vi "get-childs-tags-by-tag.vi"(8 "error in (no error)":errorcluster, 9 "tag":string, 11 "CANtable in":refnum<class "bAPPdata.lvclass">) -> (0 "error out":errorcluster, 1 "child.tags":string[](array[string]), 3 "CANtable out":refnum<class "bAPPdata.lvclass">)   [LabVIEW 2015, in "bAPPdata.lvclass"]
uses:
  bAPPdata.lvclass
  bAPPdata.lvclass/bAPPdata.ctl
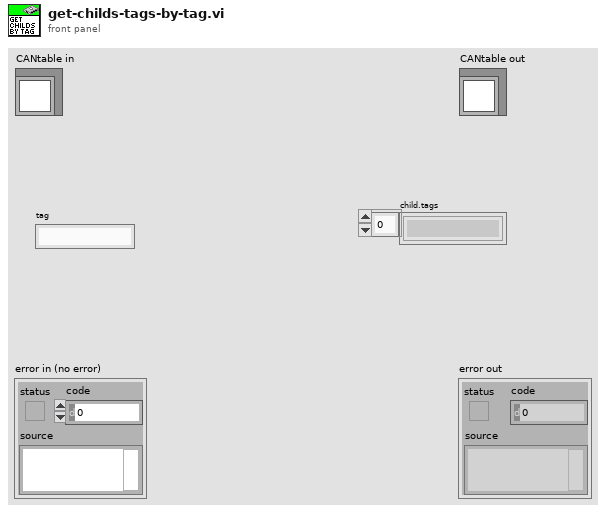
[diagram p1: front panel]
types:
  T1 = typedef "bAPPdata.lvclass/table-data.ctl" = T2[]
  T2 = typedef "bAPPdata.lvclass/table-contents.ctl" = cluster{"id":u32, "tag":string, "frame.type":T3, "last.frame":T4, "tMsgData":T6, "child.tags":string[], "bit-payload":bool[]}
  T3 = typedef "frame.type.ctl" = enum16{"FRAME NOT DEFINED", "DUT OUTPUT FRAME", "DUT INPUT FRAME"}
  T4 = typedef "XNET Frame CAN.ctl" = cluster{"timestamp":timestamp, "payload":u8[], "identifier":u32, "type":T5, "extended?":bool, "echo?":bool}
  T5 = typedef "XNET Frame Type CAN.ctl" = u8
  T6 = typedef "nMsgData.ctl" = cluster{"dwID":u32, "count":u32, "dwCycleTime":dbl, "dwTime":dbl, "new msg":bool}
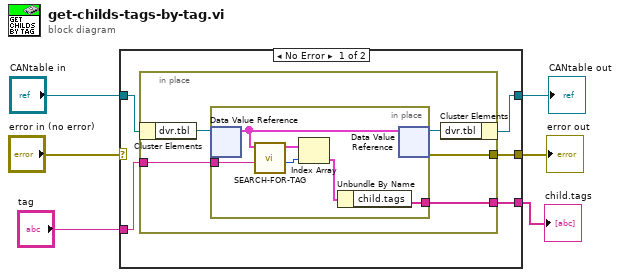
[diagram p0: block diagram]
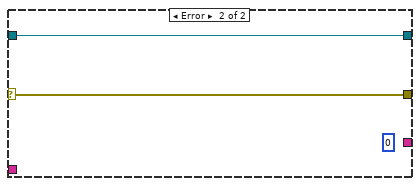
[diagram p2: hidden frame]
diagram:
  n1 = case shown="No Error" "error in (no error)" {
    selector: "error in (no error)" -> [_ w24]
    tunnel: [w9 w24] -> w5
    tunnel: [w10 w23] -> w3
    tunnel: "CANtable in" -> [w11 w23]
    tunnel: "tag" -> [w8 _]
    tunnel: [w7 _] -> w1
    frame No Error {
      n2 = in-place {
        in-place-border: [w14] -> w9
        in-place-border: w8 -> [w13]
        in-place-border: [w12] -> w7
        n3 = in-place-cluster #1(w11) -> ("dvr.tbl"=w16:refnum<data-value>)
        n4 = in-place {
          in-place-border: w13 -> [w18]
          in-place-border: [w17] -> w12
          n5 = in-place-dvr #2(w16) -> (w22:T1)  [unwired: 1 out]
          n6 = call "SEARCH-FOR-TAG.vi"("tag"=w18, "tbl.list"=w22) -> ("idx"=w21:i32, "tbl.list out"=w19:T2[])  [unwired: 8 in]
          n7 = Index Array(array=w19, index=w21) -> (element=w20:T2)
          n8 = Unbundle By Name(w20) -> ("child.tags"=w17:string[])
          n9 = in-place-dvr #2(w22) -> (w15:refnum<data-value>, w14:errorcluster)
        }
        n10 = in-place-cluster #1("dvr.tbl"=w15) -> (w10:refnum<class "bAPPdata.lvclass">)
      }
    }
    frame Error {
      (unwired) u32 0 ("id")
    }
  }
  "error out" <- w5
  "CANtable out" <- w3
  "child.tags" <- w1
